vi "DstmIO.vi"(7 "Overlap?":bool, 8 "Error In":errorcluster, 9 "Num Rec Bytes":u32, 10 "Data To Send":u8[](array[numeric]), 11 "Device Handle":u32) -> (0 "Error Out":errorcluster, 2 "Received Data":u8[](array[numeric]), 3 "Device Handle":u32)   [LabVIEW 2011, in "LVH-Adept.lvlib" / "DSTM.lvlib"]
uses:
  DSTM.lvlib
  Private/Type Defs/Error.ctl
  dstm.dll
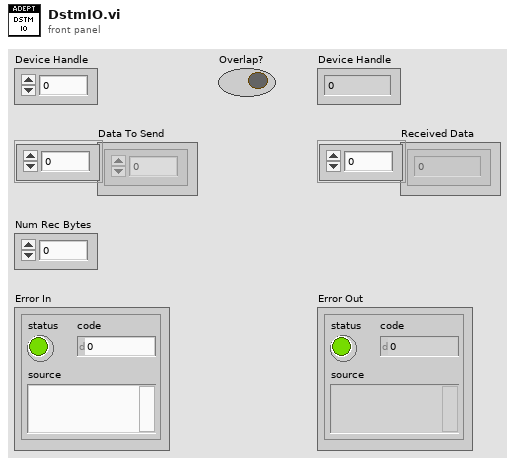
[diagram p1: front panel]
types:
  T1 = typedef "LVH-Adept.lvlib/DSTM.lvlib/Error.ctl" = enum16{"Unknown", "Enable", "Data Transfer", "Disable"}
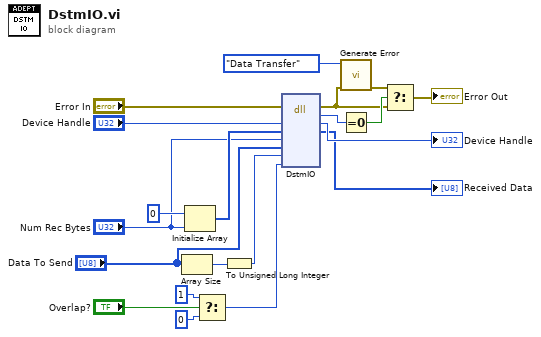
[diagram p0: block diagram]
diagram:
  n1 = Array Size(array="Data To Send") -> (size(s)=w2:i32)
  n2 = Initialize Array(u8 0, "Num Rec Bytes") -> (w10:u8[])
  n3 = Select(t=u8 1, s="Overlap?", f=u8 0) -> (s? t:f=w5:u8)
  n4 = To Unsigned Long Integer(number=w2) -> (unsigned 32bit integer=w1:u32)
  n5 = dll-call lib="dstm.dll" fn="DstmIO"(error in="Error In", "hif"="Device Handle", "rgbOut"=w10, "cbOut"="Num Rec Bytes", "rgbIn"="Data To Send", "cbIn"=w1, "fOverlap"=w5) -> (error out=w13:errorcluster, "Success"=w19:u32, "hif"=→"Device Handle":u32, "rgbOut"=→"Received Data":u8[])  [unwired: 6 in, 1 out]
  n6 = call "Generate Error.vi"("Error In"=w13, "DSTM Error"=Error."Data Transfer") -> ("Error Out"=w14:errorcluster)  [unwired: 9 in]
  n7 = Equal To 0?(x=w19) -> (x = 0?=w18:bool)
  n8 = Select(t=w14, s=w18, f=w13) -> (s? t:f=→"Error Out":errorcluster)
